vi "Event Log.vi"(8 "Message":string, 9 "Log Event Type":T1, 10 "Event Type":string, 11 "Location":string) -> ()   [LabVIEW 2024, in "Sift Stream.lvlib" / "Sift Stream.lvclass"]
doc: "Log event to log file."
uses:
  Sift Stream.lvclass
  Log Event Types.ctl
  Sift Stream.lvclass/Sift Stream.ctl
  <vilib>/Utility/LVLibp/NI_PackedLibraryUtility.lvlib
panel:
  in  "error in (no error)":errorcluster
  out "error out":errorcluster
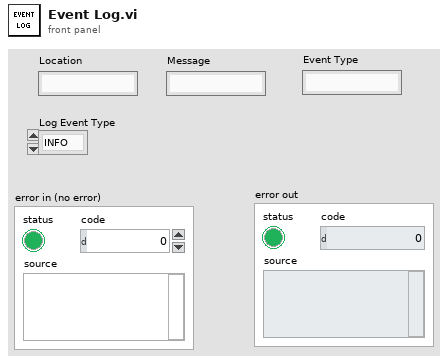
[diagram p1: front panel]
types:
  T1 = typedef "Sift Stream.lvlib/Sift Stream.lvclass/Log Event Types.ctl" = enum16{"INFO", "WARN", "ERROR"}
  T2 = enum16{"open", "replace", "create", "open or create", "replace or create", "replace or create with confirmation"}
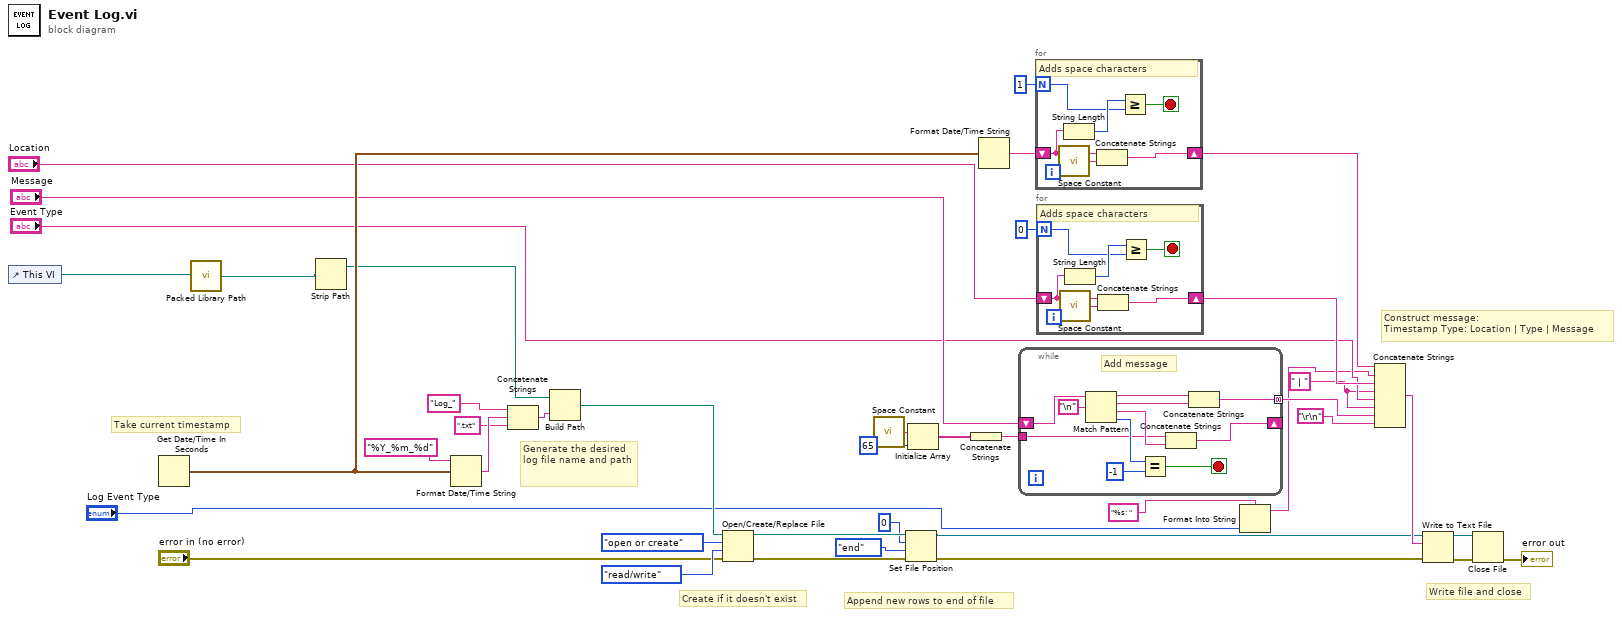
[diagram p0: block diagram]
diagram:
  w7 = " | " ("string")
  # "Write file and close"
  # "Construct message:\nTimestamp Type: Location | Type | Message"
  # "Append new rows to end of file"
  # "Create if it doesn't exist"
  # "Generate the desired log file name and path"
  # "Take current timestamp"
  n1 = control-ref of="This VI"() -> (w2:refnum<vi>)
  n2 = Get Date/Time In Seconds() -> (seconds since 1Jan1904=w14:timestamp)
  n3 = call <vilib>:"Packed Library Path.vi"("vi reference"=w2) -> ("packed library path"=w1:path)  [unwired: 2 in, 2 out]
  n4 = Strip Path(path=w1) -> (stripped path=w4:path)  [unwired: 1 out]
  n5 = Format Date/Time String(time format string (%c)="%Y_%m_%d", seconds (now)=w14) -> (date/time string=w29:string)  [unwired: 1 in]
  n6 = Concatenate Strings("Log_" ("string"), w29, ".txt" ("string")) -> (w28:string)
  n7 = Build Path(base path=w4, name or relative path=w28) -> (appended path=w15:path)
  n8 = Open/Create/Replace File(file path (use dialog)=w15, error in="error in (no error)", operation (0:open)=T2."open or create", access (0:read/write)=enum16{"read/write", "read-only", "write-only"}."read/write") -> (refnum out=w24:refnum<file>, error out=w25:errorcluster)  [unwired: 2 in, 1 out]
  n9 = call <vilib>:"Space Constant.vi"() -> ("String"=w35:string)
  n10 = Set File Position(offset (in bytes) (0)=i64 0, refnum=w24, from (0:start)=enum16{"start", "end", "current"}."end", error in=w25) -> (refnum out=w16:refnum<file>, error out=w20:errorcluster)
  n11 = Initialize Array(w35, 65 ("dimension size")) -> (w33:string[])
  n12 = Concatenate Strings(w33) -> (w32:string)
  n13 = Format Date/Time String(seconds (now)=w14) -> (date/time string=w38:string)  [unwired: 2 in]
  n14 = while {
    shift-right: [w45] -> _
    shift-left: "Message" -> [w48]
    tunnel: w32 -> [w46]
    tunnel: [w42] -> w9 mode=concatenating
    stop <- w49 stop-if-true
    # "Add message"
    n15 = Match Pattern(string=w48, regular expression="\n") -> (before substring=w44:string, match substring=w43:string, after substring=w47:string, offset past match=w50:i32)  [unwired: 1 in]
    n16 = Equal?(x=w50, y=-1) -> (x = y?=w49:bool)
    n17 = Concatenate Strings(w46, w47) -> (w45:string)
    n18 = Concatenate Strings(w44, w43) -> (w42:string)
  }
  n19 = for {
    N: 1 -> [w53]
    shift-right: [w55] -> w37
    shift-left: w38 -> [w58]
    stop <- w54 stop-if-true
    # "Adds space characters"
    n20 = call <vilib>:"Space Constant.vi"() -> ("String"=w56:string)
    n21 = String Length(string=w58) -> (length=w57:i32)
    n22 = Concatenate Strings(w58, w56) -> (w55:string)
    n23 = Greater Or Equal?(x=w57, y=w53) -> (x >= y?=w54:bool)
  }
  n24 = for {
    N: 0 -> [w59]
    shift-right: [w61] -> w36
    shift-left: "Location" -> [w64]
    stop <- w60 stop-if-true
    # "Adds space characters"
    n25 = call <vilib>:"Space Constant.vi"() -> ("String"=w62:string)
    n26 = String Length(string=w64) -> (length=w63:i32)
    n27 = Concatenate Strings(w64, w62) -> (w61:string)
    n28 = Greater Or Equal?(x=w63, y=w59) -> (x >= y?=w60:bool)
  }
  n29 = Format Into String(format string="%s: ", "Log Event Type") -> (resulting string=w3:string)  [unwired: 2 in, 1 out]
  n30 = Concatenate Strings(w37, w3, w36, w7, "Event Type", w7, w9, "\r\n") -> (w41:string)
  n31 = Write to Text File(file (use dialog)=w16, text=w41, error in=w20) -> (refnum out=w19:refnum<file>, error out=w18:errorcluster)  [unwired: 1 in, 1 out]
  n32 = Close File(refnum=w19, error in=w18) -> (error out=→"error out":errorcluster)  [unwired: 1 out]
